vi "PathGenerator.vi"(2 "error in":errorcluster, 3 "data type":variant, 4 "number":i32, 5 "Channel Array In":T1(array[cluster])) -> (0 "error out":errorcluster, 1 "Channel Array Out":T1(array[cluster]))   [LabVIEW 2014]
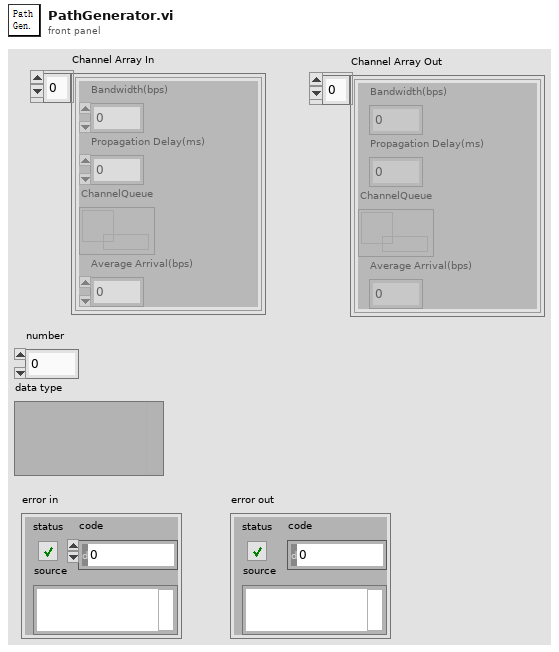
[diagram p1: front panel]
types:
  T1 = cluster{"Bandwidth(bps)":i32, "Propagation Delay(ms)":i32, "ChannelQueue":refnum<queue>, "Average Arrival(bps)":dbl}[]
  T2 = cluster{"Bandwidth(bps)":i32, "Propagation Delay(ms)":i32, "ChannelQueue":refnum<queue>, "Average Arrival(bps)":dbl}
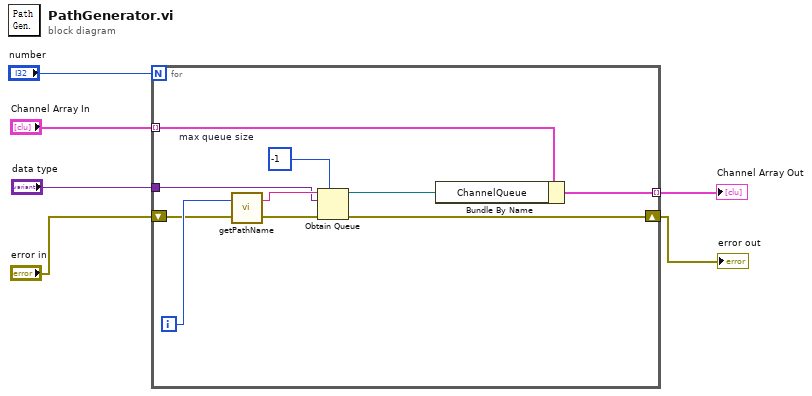
[diagram p0: block diagram]
diagram:
  n1 = for {
    N: "number" -> [_]
    shift-right: [w12] -> w3
    shift-left: "error in" -> [w11]
    tunnel: "data type" -> [w10]
    tunnel: [w8] -> w1 mode=indexing
    tunnel: "Channel Array In" -> [w7] mode=indexing
    i -> [w16]
    w13 = -1  # max queue size
    n2 = call "getPathName.vi"("error in"=w11, "No."=w16) -> ("error out"=w14:errorcluster, "resulting string"=w15:string)
    n3 = Obtain Queue(max queue size (-1, unlimited)=w13, name (unnamed)=w15, element data type=w10, error in (no error)=w14) -> (queue out=w9:refnum<queue>, error out=w12:errorcluster)  [unwired: 1 in, 1 out]
    n4 = Bundle By Name(cluster=w7, "ChannelQueue"=w9) -> (w8:T2)
  }
  "error out" <- w3
  "Channel Array Out" <- w1
